vi "Semaphore Open Acquire.vi"(7 "Timeout (ms)":i32=65535, 8 "error in":errorcluster, 11 "Name":string="LabVIEW_System_Semaphore") -> (0 "error out":errorcluster, 2 "Timed Out?":bool, 3 "TDM IO Lock":u16)   [LabVIEW 2011]
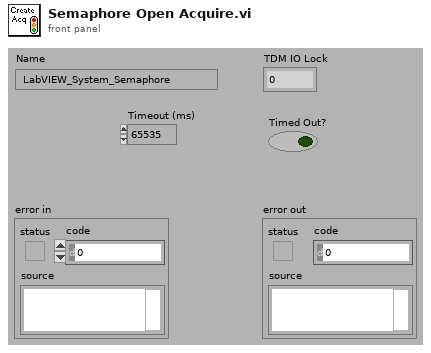
[diagram p1: front panel]
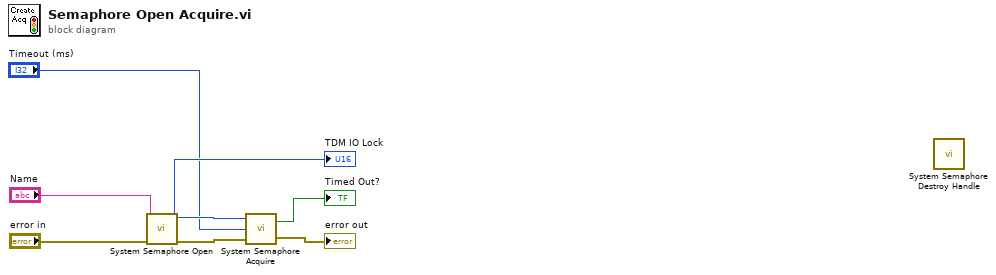
[diagram p0: block diagram]
diagram:
  n1 = call "System Semaphore Open.vi"("error in (no error)"="error in", "Name"="Name") -> ("error out"=w1:errorcluster, "Handle"=w3:u16)  [unwired: 8 in]
  "TDM IO Lock" <- w3
  n2 = call "System Semaphore Acquire.vi"("error in (no error)"=w1, "Timeout (ms)"="Timeout (ms)", "SemaphoreHandle"=w3) -> ("error out"=→"error out":errorcluster, "Timed Out?"=→"Timed Out?":bool)
  n3 = call "System Semaphore Destroy Handle.vi"() -> ()  [unwired: 11 in, 1 out]
